vi "_PC_RTLoop_Get_Sys_Log.vi"(7 "Function":enum16{"Init", "Get Data", "Close"}(ring)=enum."Close", 8 "error in (no error)":errorcluster) -> (0 "error out":errorcluster)   [LabVIEW 2018]
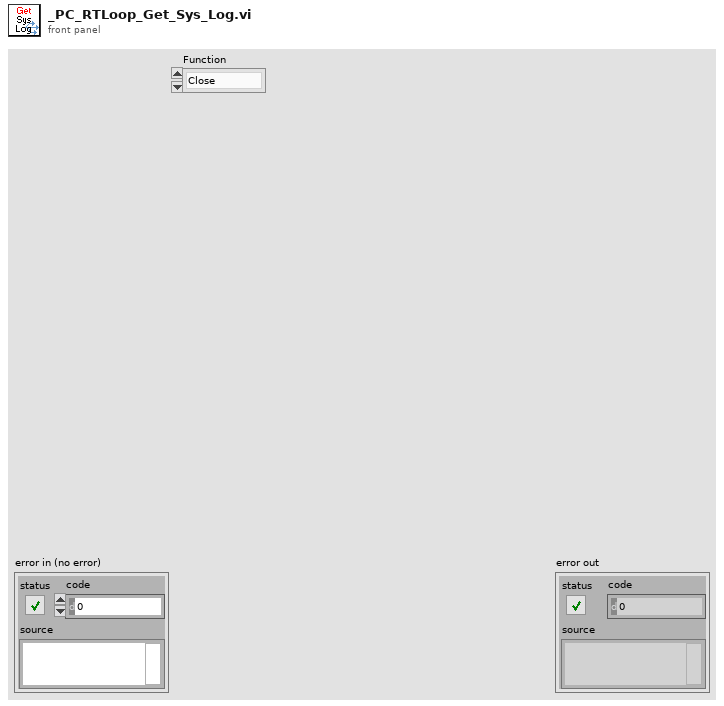
[diagram p1: front panel]
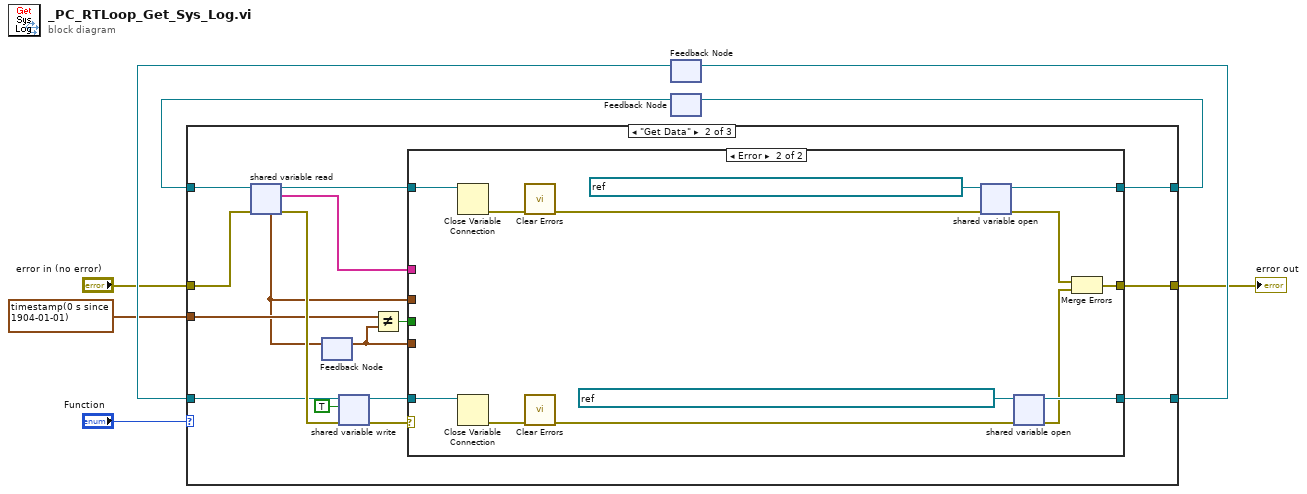
[diagram p0: block diagram]
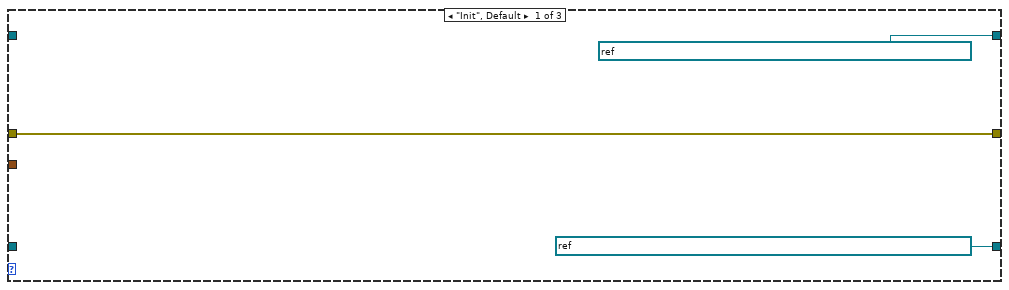
[diagram p2: hidden frame]
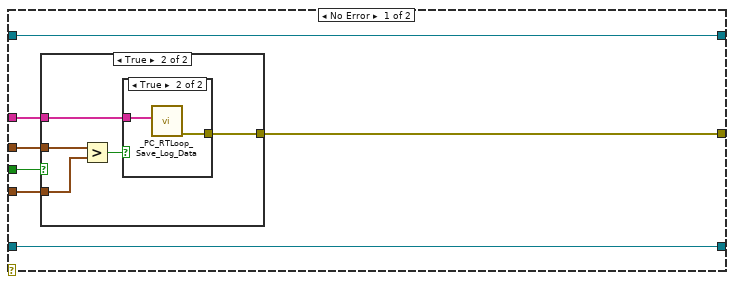
[diagram p3: hidden frame]
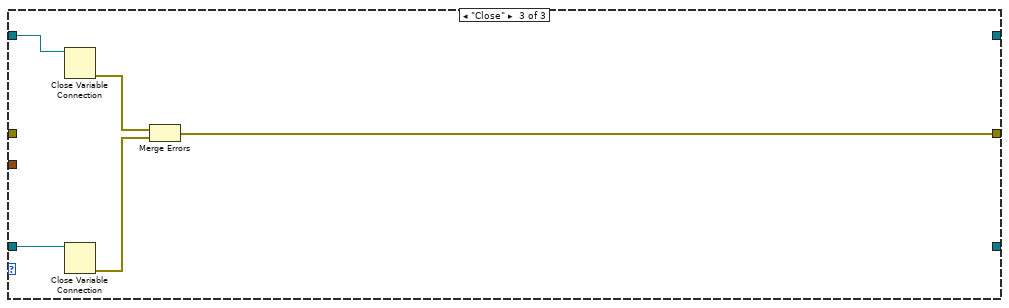
[diagram p6: hidden frame]
diagram:
  n1 = feedback #1() -> (w4:refnum<k21>)  [unwired: 1 in]
  n2 = feedback #2() -> (w6:refnum<k21>)  [unwired: 1 in]
  n3 = case shown="\"Get Data\"" "Function" {
    tunnel: [refnum<k21> "ni.var.psp://NI-sbRIO/_RT_CtrlLoop_Log_Variable/rt_log_data" ("shared variable refnum in") w13 _] -> w7
    tunnel: [refnum<k21> "ni.var.psp://NI-sbRIO/_RT_CtrlLoop_Log_Variable/rt_log_load_trigger" ("shared variable refnum in") w14 _] -> w5
    tunnel: w6 -> [_ w25 w59]
    tunnel: w4 -> [_ w24 w58]
    tunnel: "error in (no error)" -> [w9 w23 _]
    tunnel: timestamp(0 s since 1904-01-01) -> [_ w22 _]
    tunnel: [w9 w12 w55] -> w1
    frame "Init", Default {
    }
    frame "Get Data" {
      n4 = shared-variable-read(w25, w23) -> (w16:refnum<k21>, w27:errorcluster, w18:string[], w21:timestamp)
      n5 = feedback-in #3(w21) -> ()
      n6 = feedback #3() -> (w20:timestamp)  [unwired: 1 in]
      n7 = shared-variable-write(w24, w27, TRUE ("data in")) -> (w15:refnum<k21>, w17:errorcluster)
      n8 = Not Equal?(x=w22, y=w20) -> (x != y?=w19:bool)
      n9 = case shown="Error" w17 {
        tunnel: w21 -> [w34 _]
        tunnel: w20 -> [w33 _]
        tunnel: w19 -> [w32 _]
        tunnel: w18 -> [w31 _]
        tunnel: w16 -> [w29 w54]
        tunnel: w15 -> [w30 w47]
        tunnel: [w30 w46] -> w14
        tunnel: [w29 w51] -> w13
        tunnel: [w28 w42] -> w12
        frame No Error {
          n10 = case shown="True" w32 {
            tunnel: w34 -> [_ w39]
            tunnel: w33 -> [_ w38]
            tunnel: w31 -> [_ w36]
            tunnel: [_ w35] -> w28
            frame False {
            }
            frame True {
              n11 = Greater?(x=w39, y=w38) -> (0:w37:bool)
              n12 = case shown="True" w37 {
                tunnel: w36 -> [_ w41]
                tunnel: [_ w40] -> w35
                frame False {
                }
                frame True {
                  n13 = call "_PC_RTLoop_Save_Log_Data.vi"("data array of string"=w41) -> ("error out"=w40:errorcluster)  [unwired: 10 in]
                }
              }
            }
          }
        }
        frame Error {
          n14 = Close Variable Connection(11:w54) -> (0:w53:errorcluster)  [unwired: 1 in]
          n15 = Close Variable Connection(11:w47) -> (0:w48:errorcluster)  [unwired: 1 in]
          n16 = call <vilib>:"Clear Errors.vi"("error in (no error)"=w53) -> ("error out"=w50:errorcluster)  [unwired: 5 in, 1 out]
          n17 = call <vilib>:"Clear Errors.vi"("error in (no error)"=w48) -> ("error out"=w49:errorcluster)  [unwired: 5 in, 1 out]
          n18 = shared-variable-open(refnum<k21> "ni.var.psp://NI-sbRIO/_RT_CtrlLoop_Log_Variable/rt_log_data" ("shared variable refnum in"), w50) -> (w51:refnum<k21>, w44:errorcluster)
          n19 = shared-variable-open(refnum<k21> "ni.var.psp://NI-sbRIO/_RT_CtrlLoop_Log_Variable/rt_log_load_trigger" ("shared variable refnum in"), w49) -> (w46:refnum<k21>, w43:errorcluster)
          n20 = Merge Errors(w44, w43) -> (w42:errorcluster)
        }
      }
    }
    frame "Close" {
      n21 = Close Variable Connection(11:w59) -> (0:w57:errorcluster)  [unwired: 1 in]
      n22 = Close Variable Connection(11:w58) -> (0:w56:errorcluster)  [unwired: 1 in]
      n23 = Merge Errors(w57, w56) -> (w55:errorcluster)
    }
  }
  "error out" <- w1
  n24 = feedback-in #1(w5) -> ()
  n25 = feedback-in #2(w7) -> ()
